vi "Set error.vi"(8 "Error In":errorcluster, 11 "Errors":enum16{"Cal file not found"}(ring)) -> (0 "Error Out":errorcluster)   [LabVIEW 2020, in "PathControl.lvclass"]
uses:
  PathControl.lvclass
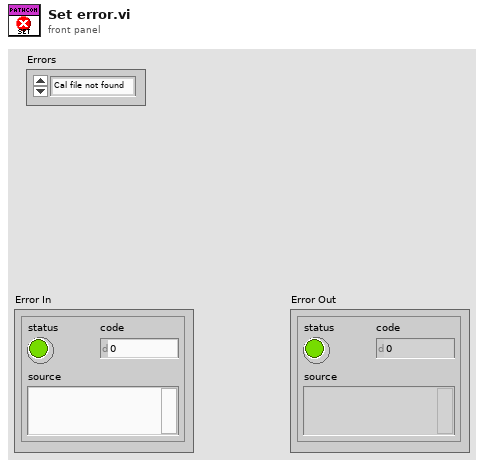
[diagram p1: front panel]
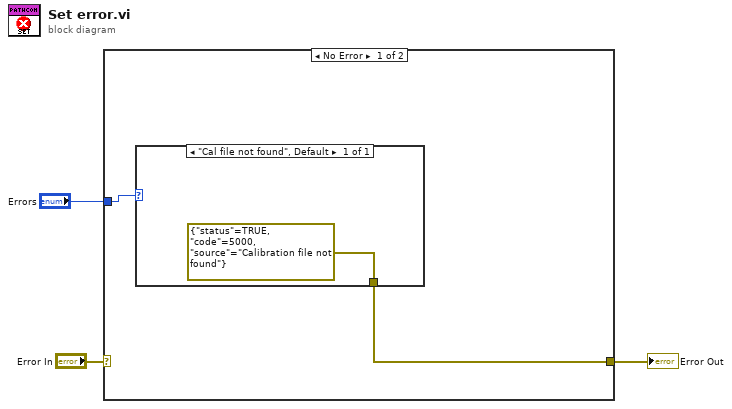
[diagram p0: block diagram]
diagram:
  n1 = case shown="No Error" "Error In" {
    selector: "Error In" -> [_ w7]
    tunnel: [w4 w7] -> w2
    tunnel: "Errors" -> [w5 _]
    frame No Error {
      n2 = case shown="\"Cal file not found\", Default" w5 {
        tunnel: [errorcluster {"status"=TRUE, "code"=5000, "source"="Calibration file not found"} ("error out")] -> w4
        frame "Cal file not found", Default {
        }
      }
    }
    frame Error {
    }
  }
  "Error Out" <- w2
